vi "HEWH Find Header.vi"(10 "Expression":string="[Uu][Pp][Pp][Ee][Rr] [Ee][Ll][Ee][Mm][Ee][Nn][Tt]", 11 "Header":string[](array[string])) -> (3 "Index":i32)   [LabVIEW 2020]
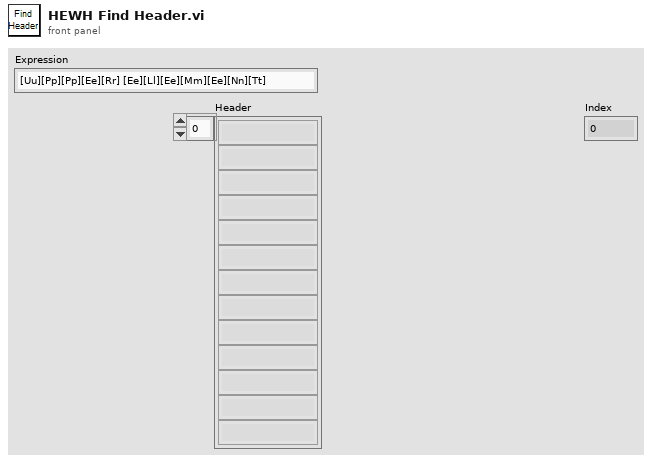
[diagram p1: front panel]
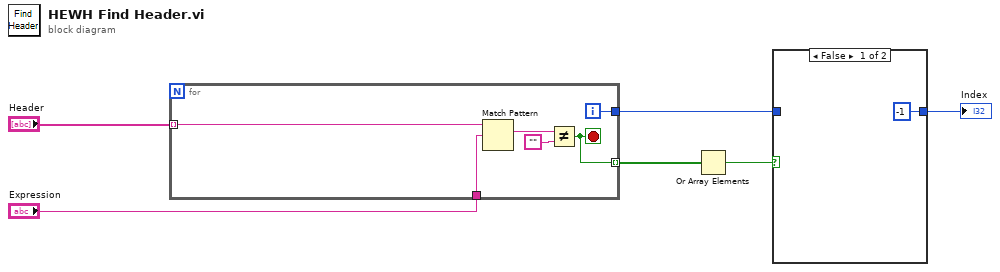
[diagram p0: block diagram]
diagram:
  n1 = for {
    tunnel: "Header" -> [w12] mode=indexing
    tunnel: [w9] -> w2
    tunnel: "Expression" -> [w8]
    tunnel: [w7] -> w4 mode=indexing
    i -> [w9]
    stop <- w7 stop-if-true
    n2 = Match Pattern(string=w12, regular expression=w8) -> (match substring=w10:string)  [unwired: 1 in, 3 out]
    n3 = Not Equal?(x=w10, y="") -> (x != y?=w7:bool)
  }
  n4 = Or Array Elements(Boolean array=w4) -> (logical OR=w3:bool)
  n5 = case shown="False" w3 {
    tunnel: w2 -> [_ w14]
    tunnel: [-1 w14] -> w1
    frame False {
    }
    frame True {
    }
  }
  "Index" <- w1
